vi "Write Playbook_v2.vi"(8 "error in (no error)":errorcluster, 10 "Playbook_v2":refnum<class "Playbook_v2.lvclass">, 11 "Game in":refnum<class "Game.lvclass">) -> (0 "error out":errorcluster, 3 "Game out":refnum<class "Game.lvclass">)   [LabVIEW 2023, in "Game.lvclass"]
uses:
  Game.lvclass
  NewSTP/Playbook_v2_class/Playbook_v2.lvclass
  Game.lvclass/Game.ctl
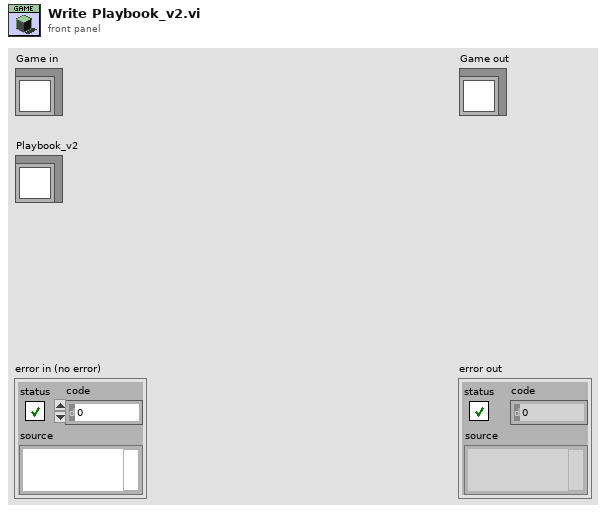
[diagram p1: front panel]
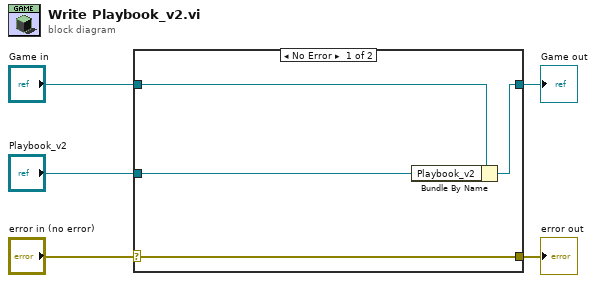
[diagram p0: block diagram]
diagram:
  n1 = case shown="No Error" "error in (no error)" {
    selector: "error in (no error)" -> [w9 w10]
    tunnel: [w9 w10] -> w4
    tunnel: [w7 w11] -> w2
    tunnel: "Game in" -> [w8 w11]
    tunnel: "Playbook_v2" -> [w6 _]
    frame No Error {
      n2 = Bundle By Name(cluster=w8, "Playbook_v2"=w6) -> (w7:refnum<class "Game.lvclass">)
    }
    frame Error {
    }
  }
  "error out" <- w4
  "Game out" <- w2
